vi "Morse Code Encoder.vi"(10 "Map":map{string, string}(c390), 11 "Message to Encode":string) -> (3 "string array":string[](array[string]))   [LabVIEW 2022 SP3]
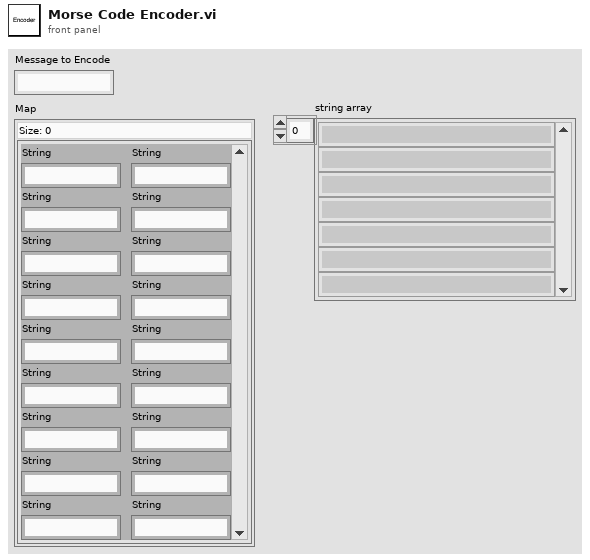
[diagram p1: front panel]
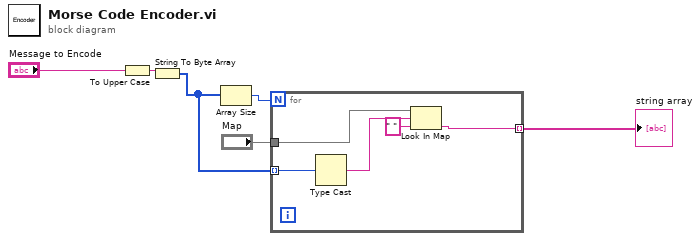
[diagram p0: block diagram]
diagram:
  n1 = To Upper Case(1:"Message to Encode") -> (0:w5:string)
  n2 = String To Byte Array(string=w5) -> (unsigned byte array=w6:u8[])
  n3 = Array Size(array=w6) -> (size(s)=w4:i32)
  n4 = for {
    N: w4 -> [_]
    tunnel: "Map" -> [w11]
    tunnel: w6 -> [w10] mode=indexing
    tunnel: [w8] -> w1 mode=indexing
    n5 = Type Cast(x=w10) -> (*(type *) &x=w9:string)  [unwired: 1 in]
    n6 = Look In Map(map=w11, key=w9, default value=" ") -> (value=w8:string)  [unwired: 1 out]
  }
  "string array" <- w1
